vi "Server.vi"() -> ()   [LabVIEW 2021]
doc: "This VI acts as a server for an incoming websockets connection. Receives/sends string data to the connected client.\nWebSockets 1.6.0.22\nSam Sharp - MediaMongrels Ltd\nCopyright (c) 2016, MediaMongrels Ltd"
uses:
  StatusCode.ctl
  Opcode.ctl
  <vilib>/Platform/browser.llb/Open URL in Default Browser (path).vi
  LV WebSockets.lvlib
panel:
  in  "Secure Server":bool
  out "Opcode out":T1
  out "Close Reason Given":bool
  in  "Client Type to Open":enum16{"Web Client", "LabVIEW Client"}(ring)=enum."LabVIEW Client"
  out "Status Code":T2=1000 items=["Normal Closure"=1000, "Going Away"=1001, "Protocol Error"=1002, "Wrong Data Type"=1003, "Reserved 1004"=1004, "Reserved 1005"=1005, "Reserved 1006"=1006, "Non Consistent Data Type"=1007, "Policy Violation"=1008, "Message Too Big"=1009, "Extensions Negotiation Error"=1010, "Unexpected Condition"=1011, "Reserved 1015"=1015]
  out "Close Reason":string
  in  "Resource Names":string[](array[string])=["/resource/name"]
  out "Host":string
  out "Resource Name":string
  out "Request URI":string
  out "HTTP Headers":variant
  in  "Stop":bool
  out "Received Data":string
  in  "Send":bool
  in  "Data":string
  # "WebSockets Example Server"
  # "This VI is a simple example of sending/receiving data using WebSockets.\nIt waits for a single incoming WebSockets connection on Port 6123 and\nthen displays incoming string data. Strings can also be sent back to the client.\n\nInstructions for use:\n1) Choose the client to be automatically opened (Web or LabVIEW client)\n2) Set suitable resource names and choose wether to secure the TCP connection (TLS)\n3) Run this VI\n4) The web client will display the status of the connection and once established, data can be sent/received from either this VI or the index.html file. The LabVIEW client has a very similar interface to the server, the user has to run it after having set a suitable resource name"
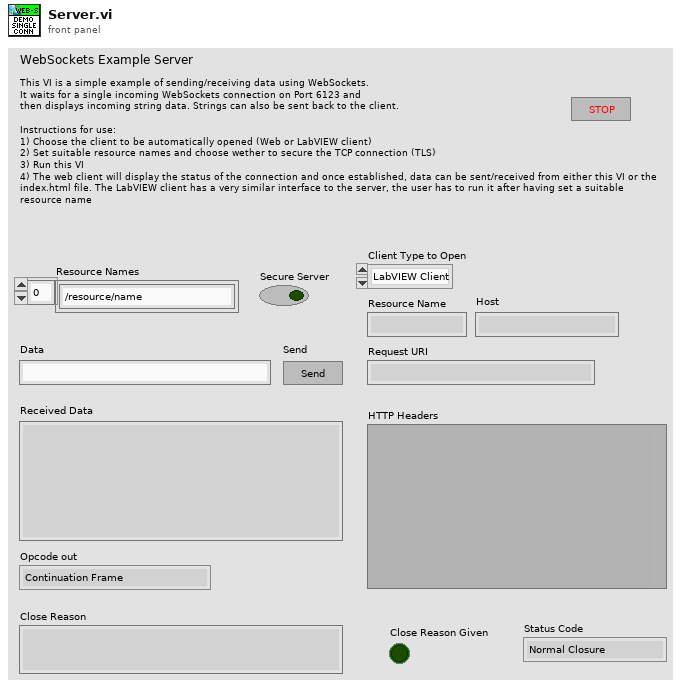
[diagram p1: front panel]
types:
  T1 = typedef "LV WebSockets.lvlib/Opcode.ctl" = enum8{"Continuation Frame", "Text Frame", "Binary Frame", "Reserved 3", "Reserved 4", "Reserved 5", "Reserved 6", "Reserved 7", "Connection Close", "Ping", "Pong", "Reserved B", "Reserved C", "Reserved D", "Reserved F"}
  T2 = typedef "LV WebSockets.lvlib/StatusCode.ctl" = u16
  T3 = enum32{"Invalid", "Standard", "Closed", "Hidden", "Minimized", "Maximized"}
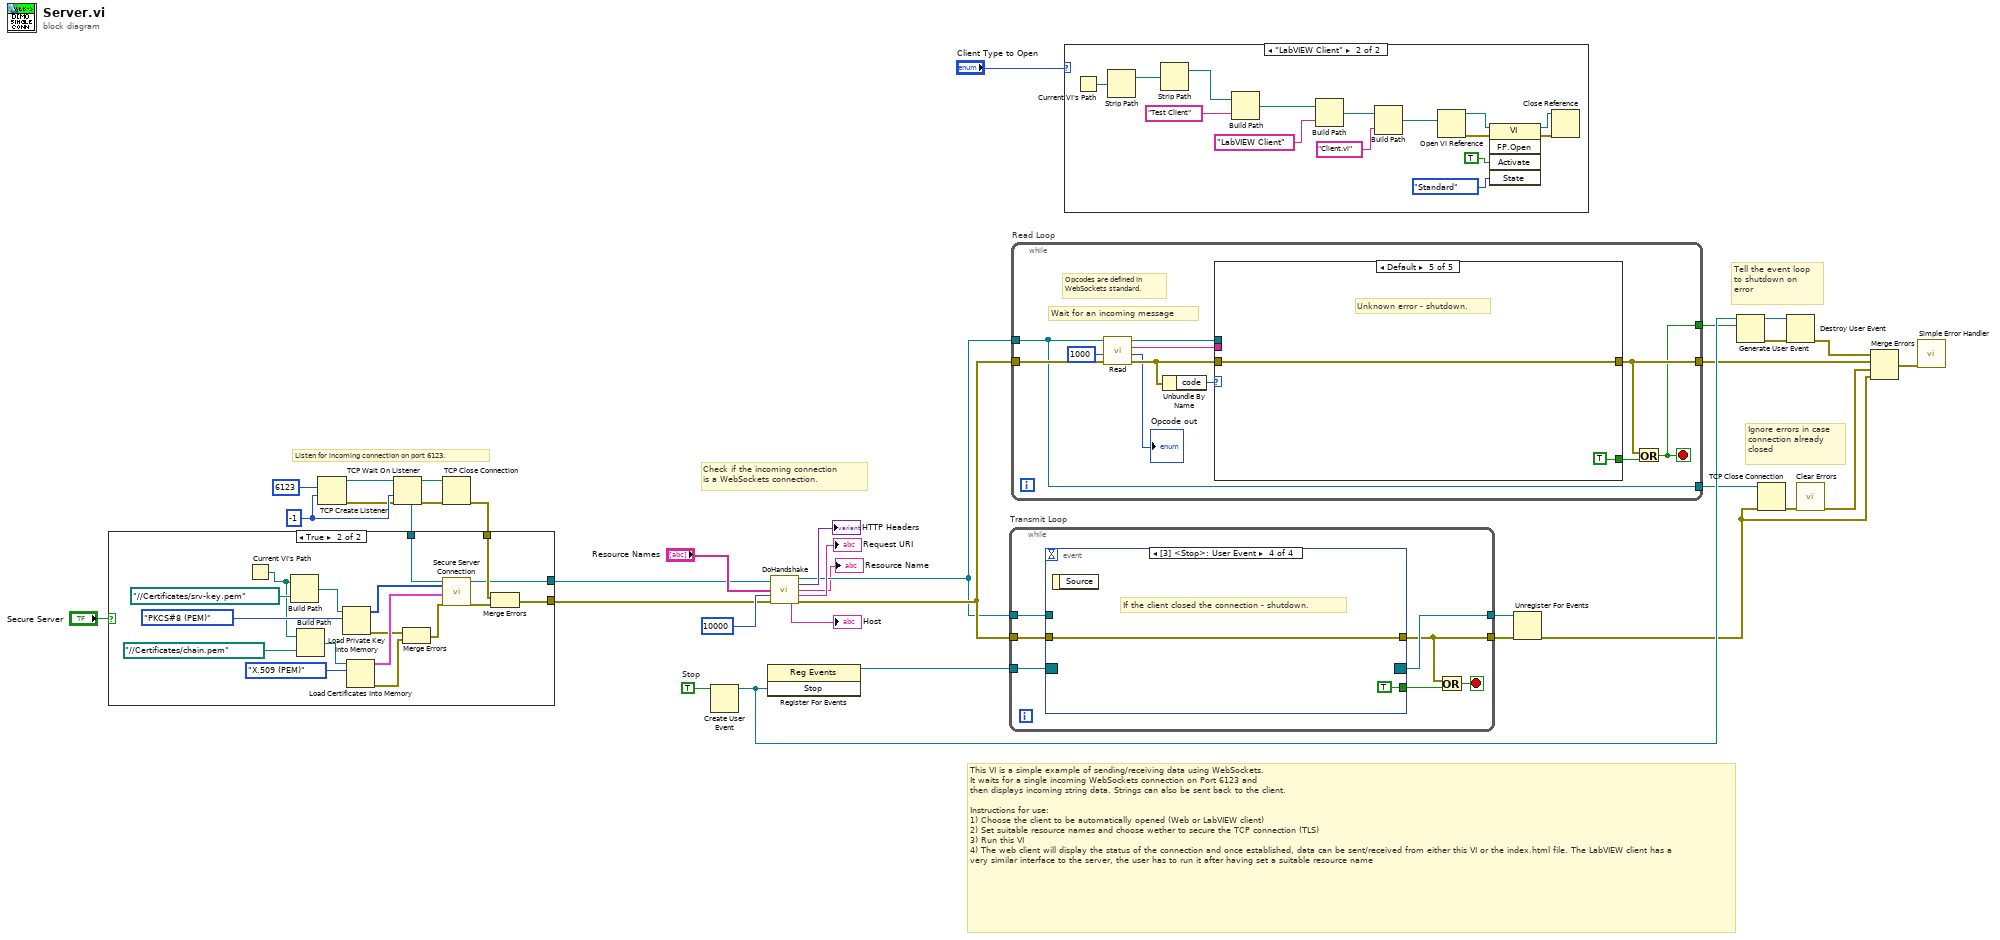
[diagram p0: block diagram]
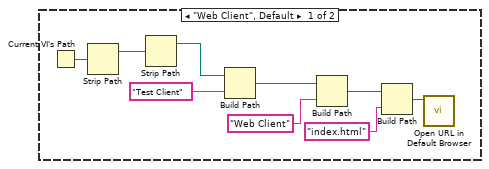
[diagram p3: hidden frame]
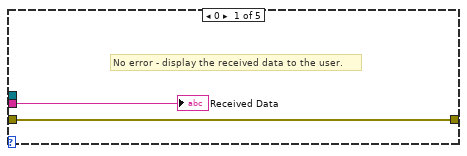
[diagram p4: hidden frame]
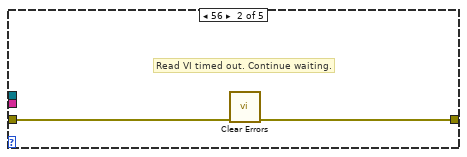
[diagram p5: hidden frame]
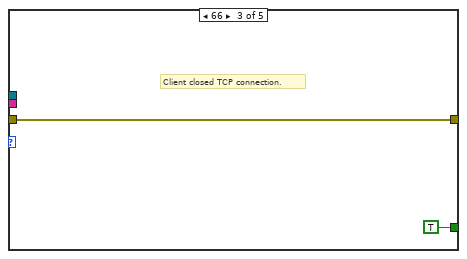
[diagram p6: hidden frame]
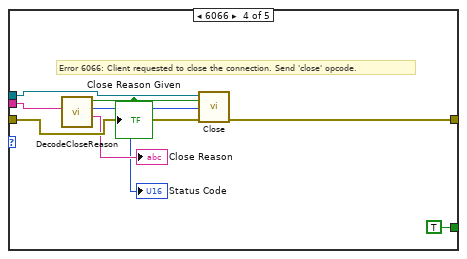
[diagram p7: hidden frame]
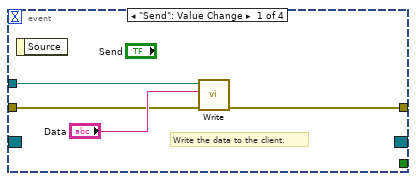
[diagram p8: hidden frame]
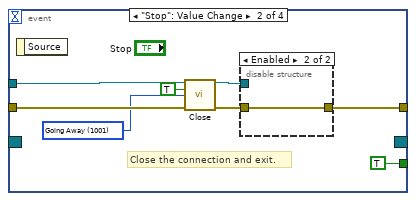
[diagram p9: hidden frame]
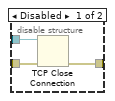
[diagram p10: hidden frame]
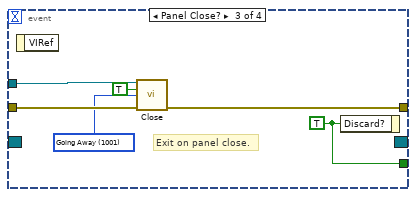
[diagram p11: hidden frame]
diagram:
  w28 = TRUE  # Stop
  w34 = -1 ("timeout ms (25000)")
  # "Ignore errors in case\nconnection already\nclosed"
  # "Tell the event loop to shutdown on error"
  # "This VI is a simple example of sending/receiving data using WebSockets.\nIt waits for a single incoming WebSockets connection on Port 6123 and\nthen displays incoming string data. Strings can also be sent back to the client.\n\nInstructions for use:\n1) Choose the client to be automatically opened (Web or LabVIEW client)\n2) Set suitable resource names and choose wether to secure the TCP connection (TLS)\n3) Run this VI\n4) The web client will display the status of the connection and once established, data can be sent/received from either this VI or the index.html file. The LabVIEW client has a very similar interface to the server, the user has to run it after having set a suitable resource name"
  # "Check if the incoming connection\nis a WebSockets connection."
  # "Listen for incoming connection on port 6123."
  n1 = TCP Create Listener(9:w34, 10:u16 6123 ("port")) -> (0:w32:errorcluster, 3:w33:refnum<k5>)  [unwired: 3 in, 1 out]
  n2 = TCP Wait On Listener(8:w32, 9:w34, 11:w33) -> (0:w30:errorcluster, 3:w31:refnum<k5>, 4:w5:refnum<k5>)  [unwired: 1 in, 2 out]
  n3 = TCP Close Connection(connection ID=w31, error in (no error)=w30) -> (error out=w12:errorcluster)  [unwired: 1 in, 1 out]
  n4 = case shown="True" "Secure Server" {
    tunnel: w12 -> [w36 w54]
    tunnel: w5 -> [w37 w45]
    tunnel: [w37 w44] -> w4
    tunnel: [w36 w43] -> w3
    frame False {
    }
    frame True {
      n5 = Current VI's Path() -> (path=w41:path)
      n6 = Build Path(base path=w41, name or relative path=path "../../Certificates/srv-key.pem" ("key")) -> (appended path=w50:path)
      n7 = Build Path(base path=w41, name or relative path=path "../../Certificates/chain.pem" ("cert chain")) -> (appended path=w48:path)
      n8 = Load Private Key Into Memory(10:enum32{"PKCS#8 (PEM)", "PKCS#8 (DER)"}."PKCS#8 (PEM)" ("format"), 11:w50) -> (0:w40:errorcluster, 3:w46:u8[])  [unwired: 2 in]
      n9 = Load Certificates Into Memory(10:enum32{"X.509 (PEM)"}."X.509 (PEM)" ("format"), 11:w48) -> (0:w38:errorcluster, 3:w47:cluster{"certificate":u8[]}[])  [unwired: 1 in]
      n10 = Merge Errors(w40, w38) -> (w39:errorcluster)
      n11 = call "Secure Server Connection.vi"("TCP connection"=w45, "private key"=w46, "certificate chain"=w47, "error in"=w39) -> ("TCP connection out"=w44:refnum<k5>, "error out"=w42:errorcluster)  [unwired: 13 in, 1 out]
      n12 = Merge Errors(w54, w42) -> (w43:errorcluster)
    }
  }
  n13 = Create User Event(user event datatype=w28) -> (user event=w26:refnum<user-event>)  [unwired: 1 in, 1 out]
  n14 = register-events(w26) -> (reference out=w29:refnum<event-registration>)  [unwired: 2 in, 1 out]
  n15 = call "DoHandshake.vi"("WebSocket Connection in"=w4, "Resource Names"="Resource Names", "timeout ms (5000)"=10000 ("timeout ms (25000)"), "error in (no error)"=w3) -> ("WebSocket Connection out"=w15:refnum<k5>, "Headers Out"=→"HTTP Headers":variant, "Resource Name"=→"Resource Name":string, "Request URI"=→"Request URI":string, "Host"=→"Host":string, "error out"=w17:errorcluster)  [unwired: 6 in]
  n16 = while "Transmit Loop" {
    tunnel: w15 -> [w61]
    tunnel: w29 -> [w60]
    tunnel: [w59] -> w27
    tunnel: [w55] -> w18
    tunnel: w17 -> [w58]
    stop <- w56 stop-if-true
    n17 = event shown="[3] <Stop>: User Event" {
      selector: w60 -> [_ _ _ _]
      dyn-events: [_ _ _ _] -> w59
      timeout: _ -> [_ _ _ _]
      tunnel: w61 -> [w65 w72 w83 _]
      tunnel: [_ TRUE w82 TRUE] -> w57
      tunnel: [w62 w70 w81 w84] -> w55
      tunnel: w58 -> [w63 w68 w80 w84]
      event "Send": Value Change {
        # "Write the data to the client."
        n18 = event-data() -> ()  [unwired: 1 in, 1 out]
        n19 = call "Write.vi"("error in (no error)"=w63, "Data"="Data", "WebSocket Connection in"=w65) -> ("error out"=w62:errorcluster)  [unwired: 7 in, 1 out]
      }
      event "Stop": Value Change {
        w67 = T2 1001 items=["Normal Closure"=1000, "Going Away"=1001, "Protocol Error"=1002, "Wrong Data Type"=1003, "Reserved 1004"=1004, "Reserved 1005"=1005, "Reserved 1006"=1006, "Non Consistent Data Type"=1007, "Policy Violation"=1008, "Message Too Big"=1009, "Extensions Negotiation Error"=1010, "Unexpected Condition"=1011, "Reserved 1015"=1015] ("Status Code")
        # "Close the connection and exit."
        n20 = event-data() -> ()  [unwired: 1 in, 1 out]
        n21 = call "Close.vi"("WebSocket Connection in"=w72, "Send Reason (F)"=TRUE, "Status Code"=w67, "error in (no error)"=w68) -> ("WebSocket Connection in"=w71:refnum<k5>, "error out"=w69:errorcluster)  [unwired: 10 in]
        n22 = disable-structure shown="Enabled" {
          disable-tunnel: w71 -> [w76 _]
          disable-tunnel: [w75 w77] -> w70
          disable-tunnel: w69 -> [w74 w77]
          frame Disabled {
            n23 = TCP Close Connection(connection ID=w76, error in (no error)=w74) -> (error out=w75:errorcluster)  [unwired: 1 in, 1 out]
          }
          frame Enabled {
          }
        }
      }
      event Panel Close? {
        w79 = T2 1001 items=["Normal Closure"=1000, "Going Away"=1001, "Protocol Error"=1002, "Wrong Data Type"=1003, "Reserved 1004"=1004, "Reserved 1005"=1005, "Reserved 1006"=1006, "Non Consistent Data Type"=1007, "Policy Violation"=1008, "Message Too Big"=1009, "Extensions Negotiation Error"=1010, "Unexpected Condition"=1011, "Reserved 1015"=1015] ("Status Code")
        w82 = TRUE ("Discard?")
        # "Exit on panel close."
        n24 = event-data() -> ()  [unwired: 1 in, 1 out]
        n25 = call "Close.vi"("WebSocket Connection in"=w83, "Send Reason (F)"=TRUE, "Status Code"=w79, "error in (no error)"=w80) -> ("error out"=w81:errorcluster)  [unwired: 10 in, 1 out]
        n26 = event-data("Discard?"=w82) -> ()  [unwired: 1 in, 1 out]
      }
      event User Event {
        # "If the client closed the connection - shutdown."
        n27 = event-data() -> ()  [unwired: 1 in, 1 out]
      }
    }
    n28 = Or(x=w55, y=w57) -> (x .or. y?=w56:bool)
  }
  n29 = while "Read Loop" {
    tunnel: w15 -> [w87]
    tunnel: [w88] -> w25
    tunnel: [w90] -> w16
    tunnel: w17 -> [w91]
    tunnel: [w87] -> w8
    stop <- w88 stop-if-true
    # "Wait for an incoming message"
    # "Opcodes are defined in\nWebSockets standard."
    n30 = call "Read.vi"("error in (no error)"=w91, "timeout ms (5000)"=1000 ("timeout ms (25000)"), "WebSocket Connection in"=w87) -> ("error out"=w92:errorcluster, "Opcode out"=→"Opcode out":T1, "Data"=w94:string, "WebSocket Connection out"=w93:refnum<k5>)  [unwired: 5 in]
    n31 = Unbundle By Name(w92) -> ("code"=w95:i32)
    n32 = case shown="Default" w95 {
      tunnel: w94 -> [w98 _ _ w106 _]
      tunnel: [_ _ TRUE TRUE TRUE] -> w89
      tunnel: w93 -> [_ _ _ w110 _]
      tunnel: w92 -> [w97 w100 w101 w108 w111]
      tunnel: [w97 w99 w101 w107 w111] -> w90
      frame 0 {
        # "No error - display the received data to the user."
        "Received Data" <- w98
      }
      frame 56 {
        # "Read VI timed out. Continue waiting."
        n33 = call <vilib>:"Clear Errors.vi"("error in (no error)"=w100) -> ("error out"=w99:errorcluster)  [unwired: 5 in, 1 out]
      }
      frame 66 {
        # "Client closed TCP connection."
      }
      frame 6066 {
        # "Error 6066: Client requested to close the connection. Send 'close' opcode."
        n34 = call "DecodeCloseReason.vi"("Data"=w106) -> ("Reason"=→"Close Reason":string, "Status Code"=w104:T2, "Close Reason Given"=w103:bool)  [unwired: 8 in]
        "Status Code" <- w104
        "Close Reason Given" <- w103
        n35 = call "Close.vi"("WebSocket Connection in"=w110, "Send Reason (F)"=w103, "Status Code"=w104, "error in (no error)"=w108) -> ("error out"=w107:errorcluster)  [unwired: 10 in, 1 out]
      }
      frame Default {
        # "Unknown error - shutdown."
      }
    }
    n36 = Or(x=w90, y=w89) -> (x .or. y?=w88:bool)
  }
  n37 = case shown="\"LabVIEW Client\"" "Client Type to Open" {
    frame "Web Client", Default {
      n38 = Current VI's Path() -> (path=w121:path)
      n39 = Strip Path(path=w121) -> (stripped path=w120:path)  [unwired: 1 out]
      n40 = Strip Path(path=w120) -> (stripped path=w119:path)  [unwired: 1 out]
      n41 = Build Path(base path=w119, name or relative path="Test Client") -> (appended path=w116:path)
      n42 = Build Path(base path=w116, name or relative path="Web Client") -> (appended path=w115:path)
      n43 = Build Path(base path=w115, name or relative path="index.html") -> (appended path=w117:path)
      n44 = call-poly <vilib>:"Open URL in Default Browser.vi"("path"=w117) -> ()  [unwired: 5 in, 2 out]
    }
    frame "LabVIEW Client" {
      n45 = Current VI's Path() -> (path=w136:path)
      n46 = Strip Path(path=w136) -> (stripped path=w135:path)  [unwired: 1 out]
      n47 = Strip Path(path=w135) -> (stripped path=w134:path)  [unwired: 1 out]
      n48 = Build Path(base path=w134, name or relative path="Test Client") -> (appended path=w132:path)
      n49 = Build Path(base path=w132, name or relative path="LabVIEW Client") -> (appended path=w131:path)
      n50 = Build Path(base path=w131, name or relative path="Client.vi") -> (appended path=w128:path)
      n51 = Open VI Reference(vi path=w128) -> (vi reference=w127:refnum<vi>, error out=w124:errorcluster)  [unwired: 5 in]
      n52 = invoke class="VI" method="FP.Open"(reference=w127, error in=w124, "Activate"=TRUE ("Activate?"), "State"=T3."Standard") -> (reference out=w123:refnum<vi>, error out=w122:errorcluster)  [unwired: 1 in, 3 out]
      n53 = Close Reference(reference=w123, error in (no error)=w122) -> ()  [unwired: 1 out]
    }
  }
  n54 = Unregister For Events(event registration refnum=w27, error in=w18) -> (error out=w6:errorcluster)
  n55 = Generate User Event(user event=w26, event data cluster=w25) -> (user event out=w24:refnum<user-event>, error out=w23:errorcluster)  [unwired: 2 in]
  n56 = TCP Close Connection(connection ID=w8, error in (no error)=w6) -> (error out=w14:errorcluster)  [unwired: 1 in, 1 out]
  n57 = Destroy User Event(user event=w24, error in=w23) -> (error out=w22:errorcluster)
  n58 = call <vilib>:"Clear Errors.vi"("error in (no error)"=w14) -> ("error out"=w7:errorcluster)  [unwired: 5 in, 1 out]
  n59 = Merge Errors(w22, w16, w7, w6) -> (w1:errorcluster)
  n60 = call <vilib>:"Simple Error Handler.vi"("error in (no error)"=w1) -> ()  [unwired: 4 in, 5 out]
